vi "Selector to Data Array.vi"(8 "error in":errorcluster, 10 "Selection":string[](array[string]), 11 "Report Viewer in":refnum<class "Report Viewer.lvclass">) -> (0 "error out":errorcluster, 3 "Report Viewer out":refnum<class "Report Viewer.lvclass">)   [LabVIEW 2023, in "Report Viewer.lvlib" / "Report Viewer.lvclass"]
uses:
  Library/Report Viewer.lvclass
  Library/Report Viewer.lvclass/Report Viewer.ctl
  Custom Controls/Data to Read.ctl
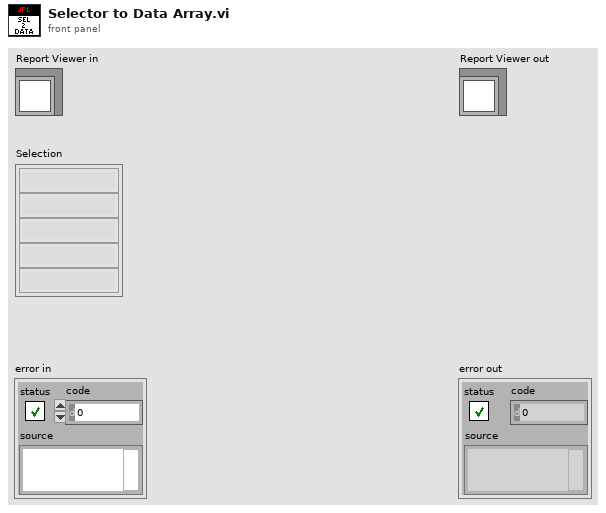
[diagram p1: front panel]
types:
  T1 = typedef "Report Viewer.lvlib/Report Viewer.lvclass/Data to Read.ctl" = cluster{"Group":string, "Channel":string}
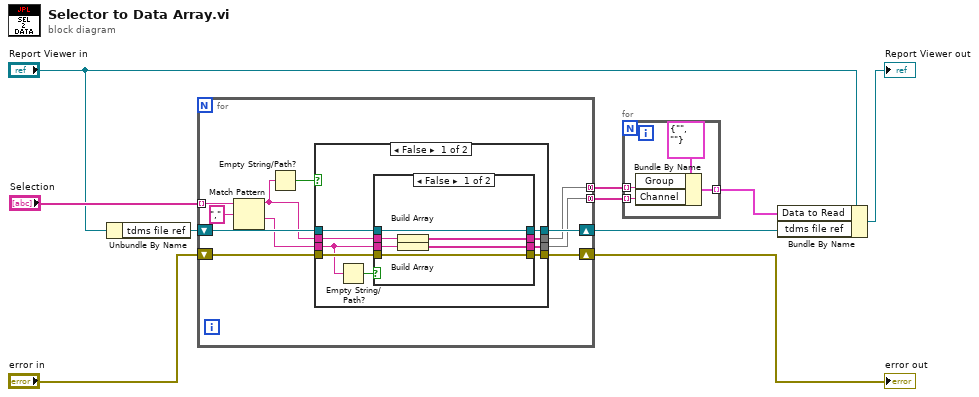
[diagram p0: block diagram]
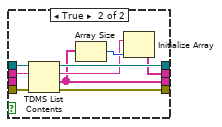
[diagram p2: hidden frame]
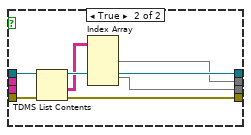
[diagram p3: hidden frame]
diagram:
  n1 = Unbundle By Name("Report Viewer in") -> ("tdms file ref"=w8:refnum<k34>)
  n2 = for {
    tunnel: "Selection" -> [w21] mode=indexing
    shift-right: [w14] -> w6
    shift-left: w8 -> [w19]
    shift-right: [w15] -> w4
    shift-left: "error in" -> [w16]
    tunnel: [w13] -> w3 mode=concatenating
    tunnel: [w12] -> w2 mode=concatenating
    n3 = Match Pattern(string=w21, regular expression=",") -> (before substring=w11:string, after substring=w17:string)  [unwired: 1 in, 2 out]
    n4 = Empty String/Path?(string/path=w11) -> (empty?=w18:bool)
    n5 = case shown="False" w18 {
      tunnel: w19 -> [w29 w52]
      tunnel: w16 -> [w28 w51]
      tunnel: w17 -> [w27 _]
      tunnel: [w26 w49] -> w15
      tunnel: [w25 w50] -> w14
      tunnel: [w24 w48] -> w12
      tunnel: w11 -> [w23 _]
      tunnel: [w22 w47] -> w13
      frame False {
        n6 = Empty String/Path?(string/path=w27) -> (empty?=w30:bool)
        n7 = case shown="False" w30 {
          tunnel: w29 -> [w35 w45]
          tunnel: w28 -> [w36 w44]
          tunnel: [w36 w43] -> w26
          tunnel: [w35 w42] -> w25
          tunnel: w23 -> [w32 w41]
          tunnel: [w33 w37] -> w24
          tunnel: w27 -> [w34 _]
          tunnel: [w31 w38] -> w22
          frame False {
            n8 = Build Array(w32) -> (w31:string[])
            n9 = Build Array(w34) -> (w33:string[])
          }
          frame True {
            n10 = TDMS List Contents(4:w44, 6:w41, 7:w45) -> (0:w43:errorcluster, 1:w37:string[], 2:w39:string, 3:w42:refnum<k34>)
            n11 = Array Size(array=w37) -> (size(s)=w40:i32)
            n12 = Initialize Array(w39, w40) -> (w38:string[])
          }
        }
      }
      frame True {
        n13 = TDMS List Contents(4:w51, 7:w52) -> (0:w49:errorcluster, 1:w46:string[][], 3:w50:refnum<k34>)  [unwired: 1 in, 1 out]
        n14 = Index Array(array=w46) -> (element #1=w47:string[], element #2=w48:string[])  [unwired: 4 in]
      }
    }
  }
  "error out" <- w4
  n15 = for {
    tunnel: w3 -> [w55] mode=indexing
    tunnel: w2 -> [w54] mode=indexing
    tunnel: [w53] -> w1 mode=indexing
    n16 = Bundle By Name(cluster=T1 {"Group"="", "Channel"=""} ("Data to read"), "Group"=w55, "Channel"=w54) -> (w53:T1)
  }
  n17 = Bundle By Name(cluster="Report Viewer in", "Data to Read"=w1, "tdms file ref"=w6) -> (→"Report Viewer out":refnum<class "Report Viewer.lvclass">)
